vi "IP_IDtoString.vi"(0 "表格引用":refnum<vi>, 2 "设备IP信息数组":T1(array[cluster]), 4 "侦听ID":refnum<k5>, 12 "不允许重复？":bool, 13 "非重复列索引":dbl) -> (19 "非新增？":bool)   [LabVIEW 2019]
panel:
  # "未使用\n\n将ID转换为字符串，填充到表格中\n根据设置选择是更新原有还是添加"
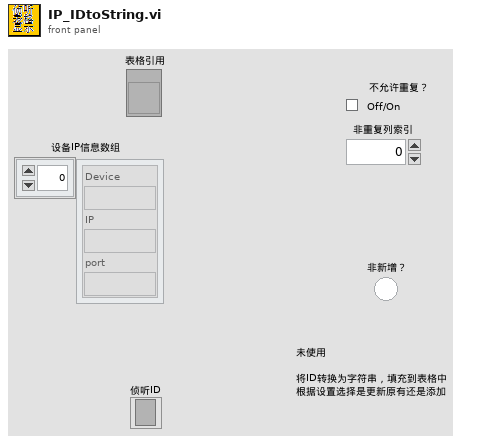
[diagram p1: front panel]
types:
  T1 = cluster{"Device":string, "IP":string, "port":string}[]
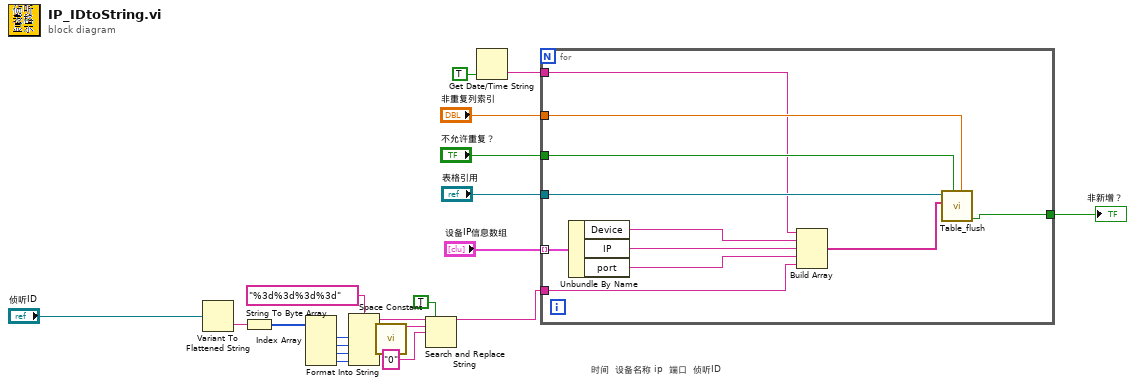
[diagram p0: block diagram]
diagram:
  # "时间  设备名称 ip  端口  侦听ID"
  n1 = Variant To Flattened String(Variant="侦听ID") -> (data string=w8:string)  [unwired: 1 out]
  n2 = String To Byte Array(string=w8) -> (unsigned byte array=w16:u8[])
  n3 = Index Array(array=w16) -> (element #1=w12:u8, element #2=w13:u8, element #3=w14:u8, element #4=w15:u8)  [unwired: 4 in]
  n4 = Format Into String(format string="%3d%3d%3d%3d" ("格式字符串"), w12, w13, w14, w15) -> (resulting string=w17:string)  [unwired: 2 in, 1 out]
  n5 = call <vilib>:"Space Constant.vi"() -> ("String"=w18:string)
  n6 = Search and Replace String(replace all?=TRUE ("替换全部？(F)"), input string=w17, search string=w18, replace string="0" ("替换字符串(\"\")")) -> (result string=w7:string)  [unwired: 4 in, 3 out]
  n7 = Get Date/Time String(want seconds? (F)=TRUE ("需要秒？(F)")) -> (time string=w19:string)  [unwired: 2 in, 1 out]
  n8 = for {
    tunnel: w19 -> [w27]
    tunnel: "设备IP信息数组" -> [w31] mode=indexing
    tunnel: "不允许重复？" -> [w30]
    tunnel: "非重复列索引" -> [w29]
    tunnel: "表格引用" -> [w28]
    tunnel: w7 -> [w22]
    tunnel: [w21] -> w1
    n9 = Unbundle By Name(w31) -> ("Device"=w26:string, "IP"=w25:string, "port"=w24:string)
    n10 = Build Array(w27, w26, w25, w24, w22) -> (w23:string[])
    n11 = call "Table_flush.vi"("唯一元素列索引"=w29, "唯一列元素？"=w30, "输入数据"=w23, "表格引用"=w28) -> ("修正重复？"=w21:bool)  [unwired: 5 in]
  }
  "非新增？" <- w1
